vi "Project Paths.vi"(11 "Project Path in":path) -> (0 "Scripts Path":path, 1 "Logs Path":path, 2 "Config Path":path, 3 "Project Path":path, 4 "Data Path":path)   [LabVIEW 2017]
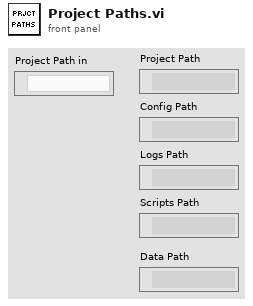
[diagram p1: front panel]
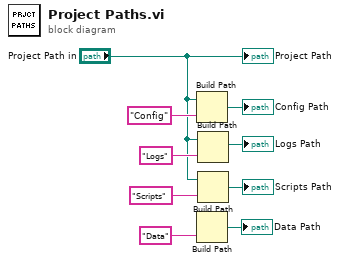
[diagram p0: block diagram]
diagram:
  n1 = Build Path(base path="Project Path in", name or relative path="Config") -> (appended path=→"Config Path":path)
  n2 = Build Path(name or relative path="Data") -> (appended path=→"Data Path":path)  [unwired: 1 in]
  n3 = Build Path(base path="Project Path in", name or relative path="Logs") -> (appended path=→"Logs Path":path)
  n4 = Build Path(base path="Project Path in", name or relative path="Scripts") -> (appended path=→"Scripts Path":path)
  "Project Path" <- "Project Path in"
